vi "Update Log Status.vi"(8 "error in (no error)":errorcluster, 11 "Waveform Log in":refnum<class "Waveform Log.lvclass">) -> (0 "error out":errorcluster, 3 "Waveform Log out":refnum<class "Waveform Log.lvclass">)   [LabVIEW 2012, in "Waveform Data Logger Engine.lvlib" / "Waveform Log.lvclass"]
uses:
  Waveform Log.lvclass
  Waveform Log.lvclass/Waveform Log.ctl
  Types/Log Status.ctl
  Waveform Data Logger Engine.lvlib
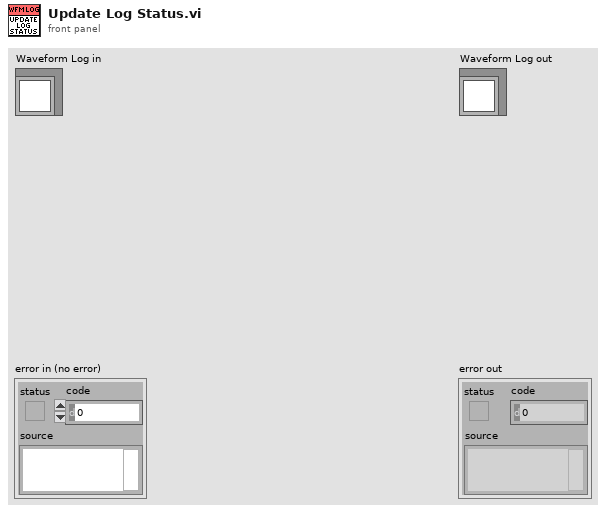
[diagram p1: front panel]
types:
  T1 = typedef "Waveform Data Logger Engine.lvlib/Log Status.ctl" = cluster{"Open Instances":i32, "Active Instances":i32, "Missed Samples":u64, "Error Code":i32}
  T2 = typedef "Waveform Data Logger Engine.lvlib/Waveform Log.lvclass/Log Instance.ctl" = cluster{"Segmented Log":refnum<data-value>, "Log Waveforms":T3[], "Log Start":timestamp, "Log Stop":timestamp, "Start Trigger Time":timestamp, "Stop Trigger Time":timestamp, "Time of Last Write":timestamp, "Timeout":dbl, "Stop cmd received":bool}
  T3 = typedef "Waveform Data Logger Engine.lvlib/Waveform Log.lvclass/Log Instance Waveform.ctl" = cluster{"Wfm Info":T4, "Count / Instance":i32, "Previous Segment":u64, "Wfm Complete?":bool, "Last Sample Logged":timestamp, "Data Logged":bool, "Log segmented":bool}
  T4 = typedef "Waveform Data Logger Engine.lvlib/Waveform Log.lvclass/Waveform Information.ctl" = cluster{"Name":string, "Wfm Data Type":T5, "Decimation":u32}
  T5 = typedef "Waveform Data Logger Engine.lvlib/Waveform Log.lvclass/Waveform Data Type.ctl" = enum16{"Double", "ComplexDouble"}
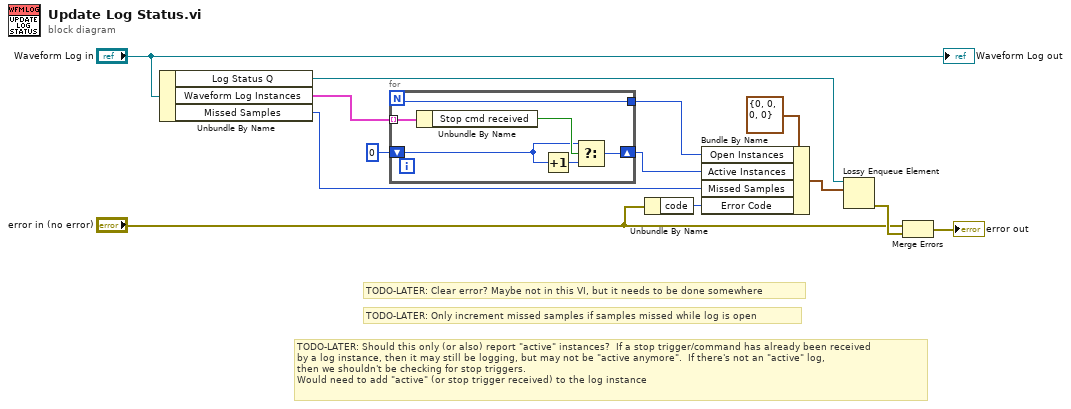
[diagram p0: block diagram]
diagram:
  # "TODO-LATER: Only increment missed samples if samples missed while log is open"
  # "TODO-LATER: Should this only (or also) report \"active\" instances?  If a stop trigger/command has already been received\nby a log instance, then it may still be logging, but may not be \"active anymore\".  If there's not an \"active\" log,\nthen we shouldn't be checking for stop triggers.\nWould need to add \"active\" (or stop trigger received) to the log instance"
  # "TODO-LATER: Clear error? Maybe not in this VI, but it needs to be done somewhere"
  n1 = Unbundle By Name("Waveform Log in") -> ("Log Status Q"=w12:refnum<queue>, "Waveform Log Instances"=w4:T2[], "Missed Samples"=w9:u64)
  n2 = for {
    N -> [w19]
    tunnel: w4 -> [w18] mode=indexing
    shift-right: [w17] -> w1
    shift-left: 0 -> [w14]
    tunnel: [w19] -> w2
    n3 = Unbundle By Name(w18) -> ("Stop cmd received"=w16:bool)
    n4 = Increment(x=w14) -> (x+1=w15:i32)
    n5 = Select(t=w14, s=w16, f=w15) -> (s? t:f=w17:i32)
  }
  n6 = Unbundle By Name("error in (no error)") -> ("code"=w10:i32)
  n7 = Bundle By Name(cluster=T1 {"Open Instances"=0, "Active Instances"=0, "Missed Samples"=0, "Error Code"=0} ("element"), "Open Instances"=w2, "Active Instances"=w1, "Missed Samples"=w9, "Error Code"=w10) -> (w5:T1)
  n8 = Lossy Enqueue Element(queue=w12, element=w5) -> (error out=w8:errorcluster)  [unwired: 1 in, 3 out]
  n9 = Merge Errors("error in (no error)", w8) -> (→"error out":errorcluster)
  "Waveform Log out" <- "Waveform Log in"
